vi "WriteStartOfRange.vi"(8 "ErrorIn":errorcluster caption="Error In(no Error)", 10 "StartOfRange":i32, 11 "ReferenceIn":refnum<class "ErrorDefinitionSQLite.lvclass"> caption="Reference In") -> (0 "ErrorOut":errorcluster caption="Error Out", 3 "ReferenceOut":refnum<class "ErrorDefinitionSQLite.lvclass"> caption="Reference Out")   [LabVIEW 2018, in "ErrorDefinitionSQLite.lvclass"]
uses:
  ErrorDefinitionSQLite.lvclass
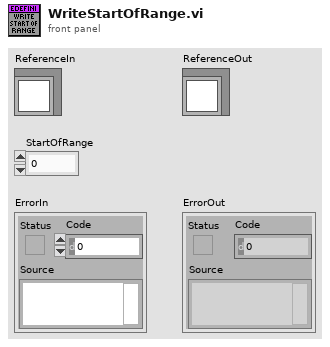
[diagram p1: front panel]
types:
  T1 = typedef "ErrorDefinitionSQLite.lvclass/ObjectAttributes.ctl" = cluster{"Path":path, "SQLiteRef":refnum<class "Connection.lvclass">, "EndOfRange":i32, "DefaultLibrarySize":i32, "StartOfRange":i32}
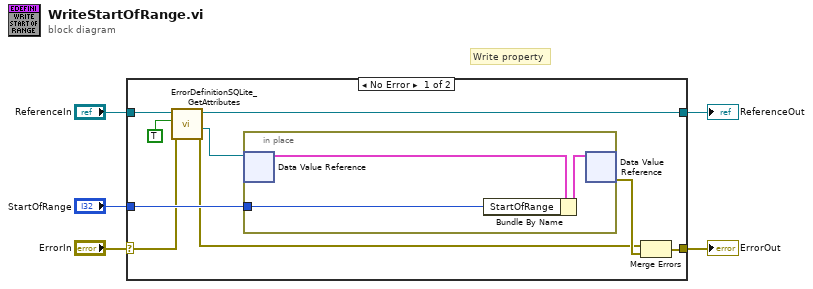
[diagram p0: block diagram]
diagram:
  # "Write property"
  n1 = case shown="No Error" "ErrorIn" {
    selector: "ErrorIn" -> [w8 w19]
    tunnel: [w12 w19] -> w4
    tunnel: [w10 w18] -> w2
    tunnel: "ReferenceIn" -> [w11 w18]
    tunnel: "StartOfRange" -> [w14 _]
    frame No Error {
      n2 = call "ErrorDefinitionSQLite_GetAttributes.vi"("ErrorIn"=w8, "OnlyGetDVRReference"=TRUE ("OnlyGetDvrReference(False)"), "Reference in"=w11) -> ("ErrorOut"=w7:errorcluster, "DataRef"=w9:refnum<data-value>, "Reference out"=w10:refnum<class "ErrorDefinitionSQLite.lvclass">)  [unwired: 5 in, 1 out]
      n3 = in-place {
        in-place-border: w14 -> [w17]
        n4 = in-place-dvr #1(w9) -> (w16:T1)  [unwired: 1 out]
        n5 = Bundle By Name(cluster=w16, "StartOfRange"=w17) -> (w15:T1)
        n6 = in-place-dvr #1(w15) -> (w13:errorcluster)  [unwired: 1 out]
      }
      n7 = Merge Errors(w7, w13) -> (w12:errorcluster)
    }
    frame Error {
    }
  }
  "ErrorOut" <- w4
  "ReferenceOut" <- w2
